vi "Pre Launch Init.vi"(11 "Histogram in":refnum<class "Histogram.lvclass">) -> (0 "error out":errorcluster, 3 "Histogram out":refnum<class "Histogram.lvclass">)   [LabVIEW 2016, in "Tests.lvlib" / "Histogram.lvclass"]
doc: "Creates neccessary user events for the Histogram Actors which can be triggered via messages"
uses:
  Histogram.lvclass
  <vilib>/vision/Image Controls.llb/IMAQ Image.ctl
  Histogram.lvclass/Histogram.ctl
  Tests.lvclass
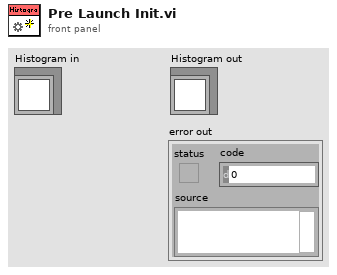
[diagram p1: front panel]
types:
  T1 = typedef "IMAQ Image.ctl" = refnum<image>
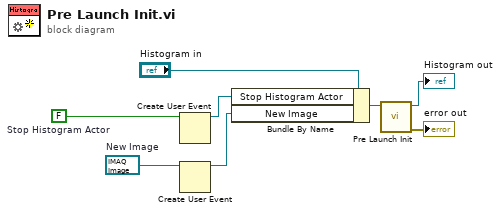
[diagram p0: block diagram]
diagram:
  w5 = T1 refnum  # New Image
  w6 = FALSE  # Stop Histogram Actor
  n1 = Create User Event(user event datatype=w6) -> (user event=w4:refnum<user-event>)  [unwired: 1 in, 1 out]
  n2 = Create User Event(user event datatype=w5) -> (user event=w3:refnum<user-event>)  [unwired: 1 in, 1 out]
  n3 = Bundle By Name(cluster="Histogram in", "Stop Histogram Actor"=w4, "New Image"=w3) -> (w1:refnum<class "Histogram.lvclass">)
  n4 = call-parent "Pre Launch Init.vi"("Actor in"=w1) -> ("error out"=→"error out":errorcluster, "Actor out"=→"Histogram out":refnum<class "Histogram.lvclass">)  [unwired: 9 in]
